vi "GetSerialNumberList.vi"() -> (1 "C400 Serial Number Array":string[](array[string]))   [LabVIEW 2017]
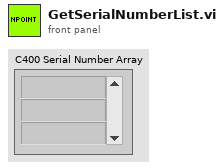
[diagram p1: front panel]
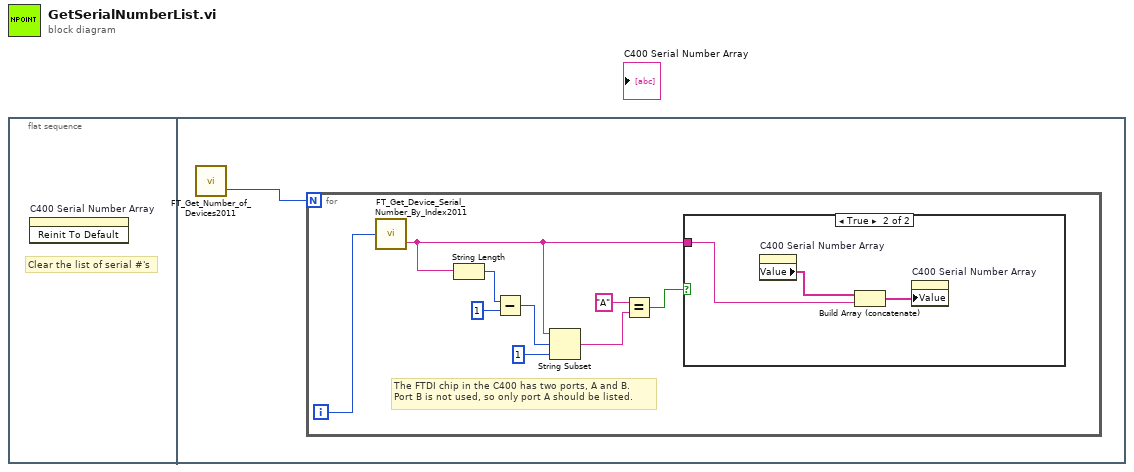
[diagram p0: block diagram]
diagram:
  n1 = flat-sequence {
    frame #0 {
      # "Clear the list of serial #'s"
      n2 = invoke on="C400 Serial Number Array" class="Arr (strict)" method="Reinit To Default"() -> ()  [unwired: 3 in, 3 out]
    }
    frame #1 {
      n3 = call "FT_Get_Number_of_Devices2011.vi"() -> ("Number of Devices"=w1:u16)  [unwired: 1 out]
      n4 = for {
        N: w1 -> [_]
        i -> [w10]
        # "The FTDI chip in the C400 has two ports, A and B.\nPort B is not used, so only port A should be listed."
        n5 = call "FT_Get_Device_Serial_Number_By_Index2011.vi"("Device Index"=w10) -> ("Device Serial Number"=w2:string)  [unwired: 1 out]
        n6 = String Length(string=w2) -> (length=w8:i32)
        n7 = Subtract(x=w8, y=1) -> (x-y=w6:i32)
        n8 = String Subset(string=w2, offset (0)=w6, length (rest)=1 ("length (rest)")) -> (substring=w5:string)
        n9 = Equal?(x="A", y=w5) -> (x = y?=w3:bool)
        n10 = case shown="True" w3 {
          tunnel: w2 -> [_ w13]
          frame False {
          }
          frame True {
            n11 = property on="C400 Serial Number Array" class="Arr (strict)"() -> ("Value"=w12:string[])  [unwired: 2 in, 2 out]
            n12 = Build Array (concatenate)(w12, w13) -> (w11:string[])
            n13 = property on="C400 Serial Number Array" class="Arr (strict)"("Value"=w11) -> ()  [unwired: 2 in, 2 out]
          }
        }
      }
    }
  }
